vi "GetText.vi"(8 "error in":errorcluster, 11 "System Diagnostics editor node in":refnum<class "System Diagnostics editor node.lvclass">) -> (0 "error out":errorcluster, 1 "additional text":string, 2 "text":string, 3 "System Diagnostics editor node out":refnum<class "System Diagnostics editor node.lvclass">, 4 "glyph":string)   [LabVIEW 2013, in "System Diagnostics editor node.lvclass"]
uses:
  System Diagnostics editor node.lvclass
  <vilib>/NI/Tag Bus Data Framework/control module/editor node/control module editor.lvclass
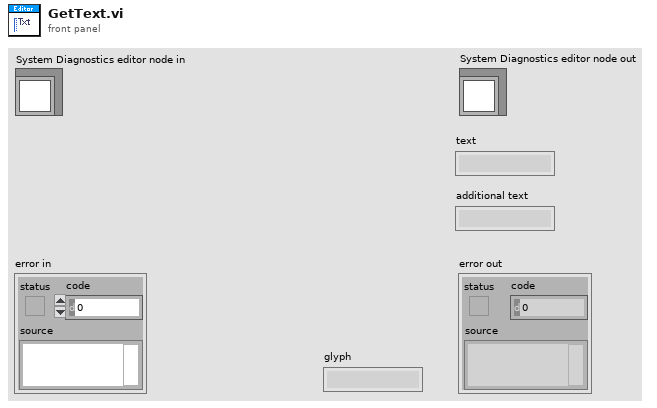
[diagram p1: front panel]
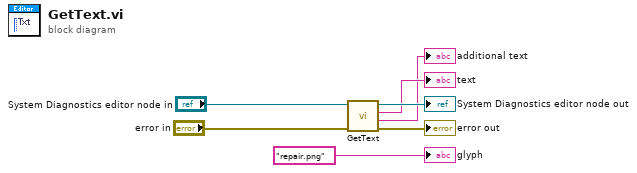
[diagram p0: block diagram]
diagram:
  n1 = call-parent "GetText.vi"("error in"="error in", "Module Editor Node in"="System Diagnostics editor node in") -> ("error out"=→"error out":errorcluster, "additional text"=→"additional text":string, "text"=→"text":string, "Module Editor Node out"=→"System Diagnostics editor node out":refnum<class "System Diagnostics editor node.lvclass">)  [unwired: 5 in, 1 out]
  "glyph" <- "repair.png" ("glyph")
